vi "Handle Remote Command.vi"(8 "error in (no error)":errorcluster, 9 "Data":string, 10 "Command":string, 11 "Example Instrument in":refnum<class "Example Instrument.lvclass">) -> (0 "error out":errorcluster, 2 "String":string, 3 "Example Instrument out":refnum<class "Example Instrument.lvclass">)   [LabVIEW 2016, in "Example Instrument.lvclass"]
uses:
  Example Instrument.lvclass
  Instrument/Instrument.lvclass
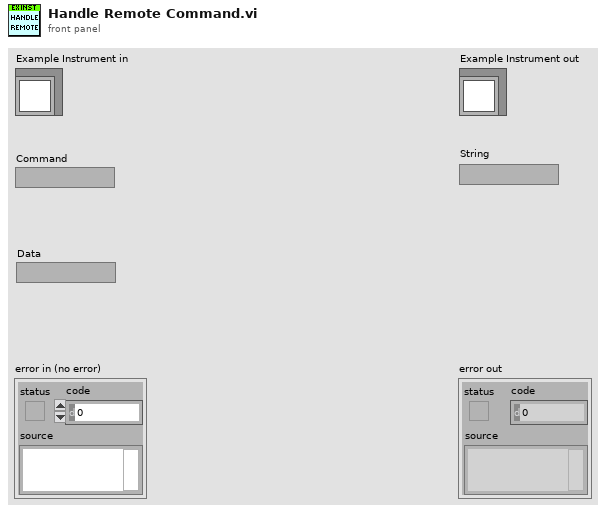
[diagram p1: front panel]
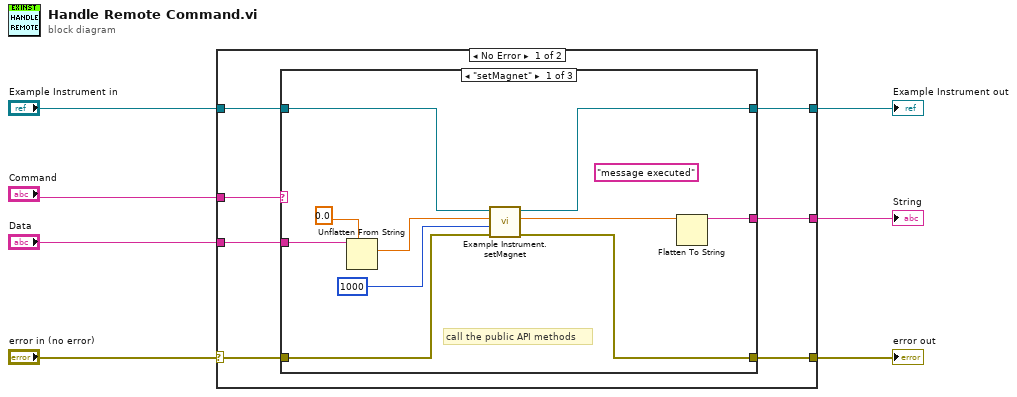
[diagram p0: block diagram]
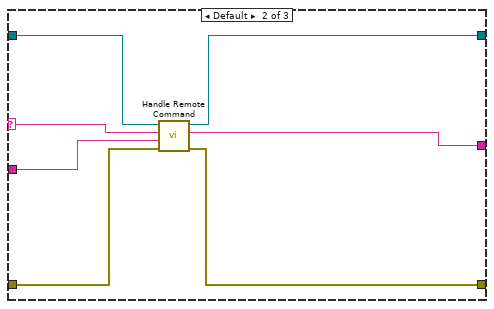
[diagram p2: hidden frame]
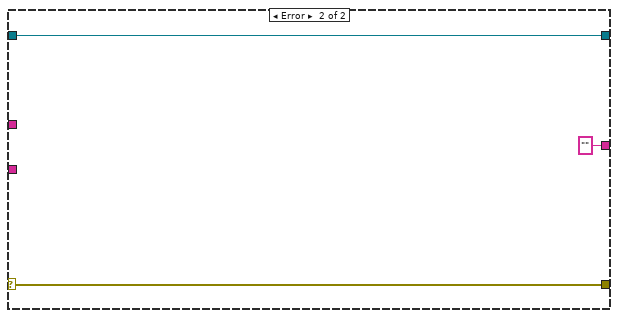
[diagram p4: hidden frame]
diagram:
  n1 = case shown="No Error" "error in (no error)" {
    selector: "error in (no error)" -> [w10 w37]
    tunnel: [w9 w37] -> w4
    tunnel: [w12 w36] -> w2
    tunnel: "Example Instrument in" -> [w13 w36]
    tunnel: "Command" -> [w14 _]
    tunnel: [w11 "" ("String")] -> w3
    tunnel: "Data" -> [w8 _]
    frame No Error {
      n2 = case shown="\"setMagnet\"" w14 {
        selector: w14 -> [_ w31 w33]
        tunnel: w13 -> [w24 w28 w32]
        tunnel: [w23 w25 w32] -> w12
        tunnel: [w15 w26 w33] -> w11
        tunnel: w10 -> [w22 w29 w34]
        tunnel: [w21 w27 w34] -> w9
        tunnel: w8 -> [w20 w30 _]
        frame "setMagnet" {
          (unwired) "message executed"
          # "call the public API methods"
          n3 = Unflatten From String(type=0.0, binary string=w20) -> (value=w18:dbl)  [unwired: 3 in, 2 out]
          n4 = call "Example Instrument.setMagnet.vi"("error in (no error)"=w22, "timeout in ms (1000)"=1000, "setMagnet"=w18, "Example Instrument"=w24) -> ("error out"=w21:errorcluster, "notification"=w16:dbl, "Example Instrument out"=w23:refnum<class "Example Instrument.lvclass">)  [unwired: 4 in, 1 out]
          n5 = Flatten To String(anything=w16) -> (data string=w15:string)  [unwired: 3 in, 2 out]
        }
        frame Default {
          n6 = call-parent "Handle Remote Command.vi"("error in (no error)"=w29, "Data"=w30, "Command"=w31, "Instrument in"=w28) -> ("error out"=w27:errorcluster, "String"=w26:string, "Instrument out"=w25:refnum<class "Example Instrument.lvclass">)  [unwired: 5 in]
        }
        frame "orlando" {
        }
      }
    }
    frame Error {
    }
  }
  "error out" <- w4
  "Example Instrument out" <- w2
  "String" <- w3
